vi "RTG_Host_Main.vi"() -> ()   [LabVIEW 2020]
uses:
  <vilib>/RTG/API/interface/public/State.ctl
  <vilib>/RTG/API/ip/common/host-types/Target Configuration.ctl
  <vilib>/RTG/API/ip/common/host-types/Synchronization - Host.ctl
  <vilib>/RTG/API/ip/common/host-types/Synchronization Mode - Host.ctl
  <vilib>/RTG/API/ip/common/host-types/Basic Target - Host.ctl
  <vilib>/RTG/API/ip/common/host-types/Target Motion Parameters.ctl
  <vilib>/RTG/API/ip/common/host-types/Single Target Motion Parameters.ctl
  <vilib>/RTG/API/interface/public/Coprocessor Link Status.ctl
  <vilib>/RTG/coprocessor/host/RTG Coprocessor Link Interface/Public/Coprocessor Status.ctl
  Controls/Enum/Program_Status_Enum.ctl
  Controls/Enum/RTG_Enum.ctl
  Controls/Enum/CoProcessor_Enum.ctl
  Controls/Enum/Supervisor_Enum.ctl
  Controls/Clust/RTG Clust.ctl
  <vilib>/RTG/API/interface/NI-RTG Interface.lvclass
  Controls/Clust/CoProcessor Clust.ctl
  <vilib>/RTG/coprocessor/host/RTG Coprocessor Link Interface/RTG Coprocessor Link Interface.lvclass
  Controls/Clust/RTG API Clust.ctl
  support/Options - API Mode.ctl
  support/Options - Calibration.ctl
  support/Options - Remote.ctl
  <vilib>/Utility/error.llb/Error Cluster From Error Code.vi
  <vilib>/rvi/errors/niLvFpgaAdjustHostInterfaceError.vi
  <vilib>/rvi/interface/nirviReadWriteControl/nirviReadWriteControl.xnode
  RTG Examples.lvlib
  <vilib>/RTG/API/ip/common/host-types/Host Data Types v1.lvlib
  NiFpgaLv.dll
  <vilib>/rvi/interface/Simulation/niFpgaSimulationCallBeginRW.vi
panel:
  out "CoPr":i32
  out "RTG":i32
  out "Spvsr":i32
  out "Spvsr":T1=enum."Spvsr_InitCtrls"
  out "CoPr":T2
  out "RTG":T3
  out "App Status":T4
  in  "Tab Control":T5(tab)
  in  "Instrument Names":string[](array[string])=["5831_0"]
  in  "Coprocessor Names":string[](array[string])
  in  "Center Freqeuncies (Hz)":dbl[](array[numeric])=[5500000000.0] format="%#_6p"
  in  "Reference Levels (dBm)":dbl[](array[numeric])=[0.0]
  in  "Calibrate":bool=TRUE
  in  "abort system self cal":bool
  in  "Commit HW":bool
  in  "ExtAtten":dbl[](array[numeric]) caption="External Attenuations (dB)"
  in  "OffsFreq":dbl[](array[numeric]) caption="Offset Frequencies (Hz)" format="%#_6p"
  in  "ExtDelay":dbl[](array[numeric]) caption="External Delay (s)" format="%#_6p"
  in  "mmWave Radio Heads Enable":bool[](array[boolean])
  in  "PRI (s)":dbl[](array[numeric]) format="%#_6p"
  in  "Set PRIs":bool
  out "Min Latencies (s)":dbl[](array[numeric]) format="%#_6p"
  out "Min Common Attenuations (dB)":dbl[](array[numeric])
  out "Max Common Attenuations (dB)":dbl[](array[numeric])
  out "Versions":string[](array[string])
  in  "Common Attenuation (dB)":dbl
  in  "Auto Send Software Trigger":bool
  in  "Prepend Software Trigger":bool
  in  "Device Index":i32
  in  "Target Configuration Files":path[](array[path])
  in  "Target Configuration":T6 {"rtg targets"."time offset (s)" format="%#_6p"; "rtg targets"."doppler" format="%#_6p"}
  in  "Target Motion Parameters":T10={"target motions"=[{"target enable"=FALSE, "start time offset (s)"=-1e-09, "time offset rate of change (s/s)"=0.001, "start attenuation (dB)"=0.0, "attenuation rate of change (dB/s)"=0.0, "start frequency shift (Hz)"=0.0, "frequency shift rate of change (Hz/sec)"=0.0}], "scenario duration (s)"=67.0, "configuration update rate(Hz)"=15000.0} {"configuration update rate(Hz)" format="%#_6p"; "target motions"."frequency shift rate of change (Hz/sec)" format="%#_6p"; "target motions"."start frequency shift (Hz)" format="%#_6p"; "target motions"."time offset rate of change (s/s)" format="%#_6p"; "target motions"."start time offset (s)" format="%#_6p"}
  in  "Send TrgtCfg":bool
  in  "Send Motion":bool
  in  "Send Files":bool
  in  "Start RTG":bool
  in  "Stop RTG":bool
  in  "Send SW Trigg":bool
  out "rtg link status":T12[](array[typedef])
  out "Trigger Count":i32[][](array[numeric]) caption="Device Index vs Trigger Count"
  out "RTG Status":string
  out "RTG State":T13
  out "error out":errorcluster
  out "System Time":string
  out "coproc link":T14[](array[typedef]) caption="coprocessor link status"
  in  "Exit":bool
  # "v20230901"
  # "Configuration Files and Target Motion"
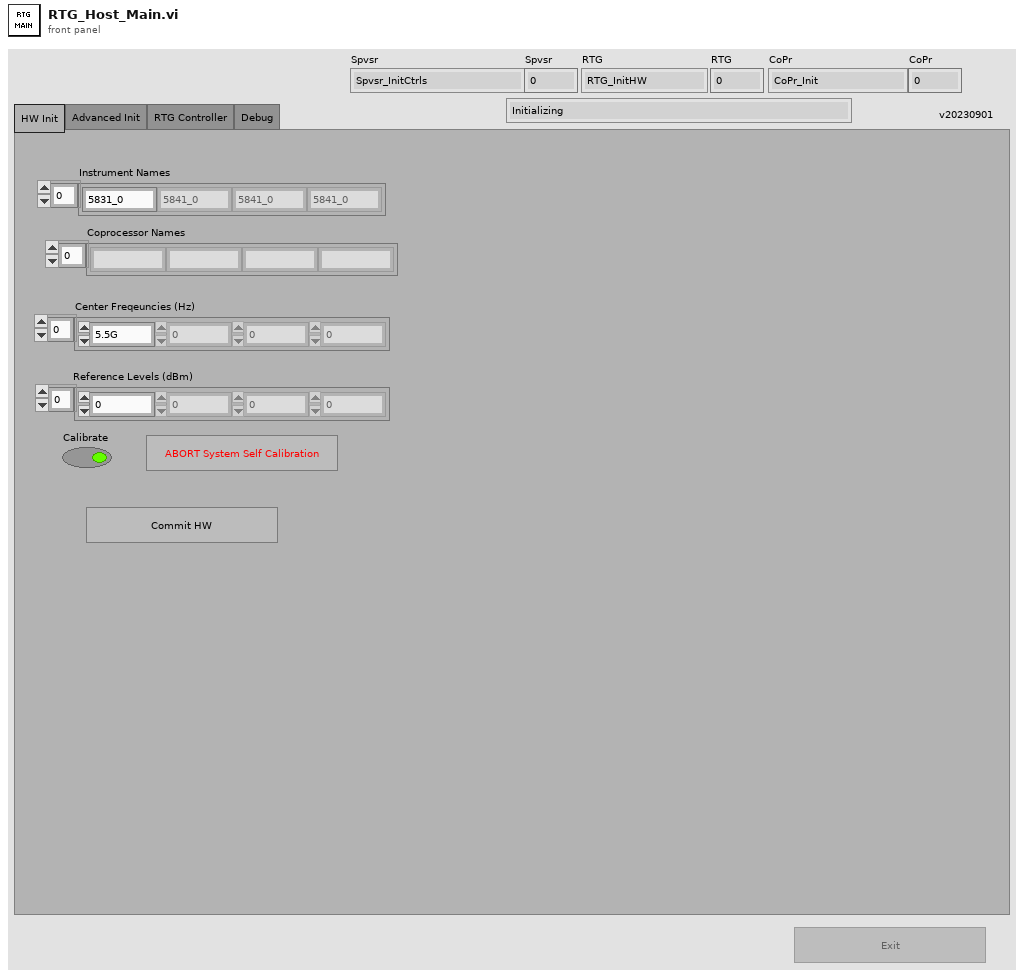
[diagram p1: front panel]
types:
  T1 = typedef "Supervisor_Enum.ctl" = enum16{"Spvsr_InitSW", "Spvsr_InitCtrls", "Spvsr_UpdtFP", "Spvsr_InitRTG", "Spvsr_StateCount", "Spvsr_Exit"}
  T2 = typedef "CoProcessor_Enum.ctl" = enum16{"CoPr_Init", "CoPr_Chk", "CoPr_Exit"}
  T3 = typedef "RTG_Enum.ctl" = enum16{"RTG_InitHW", "RTG_RefLvl", "RTG_mmWav", "RTG_Cal", "RTG_CalDone?", "RTG_ExtAtten", "RTG_GetCal", "RTG_SetPRIs", "RTG_CommAtten", "RTG_TargetSetup", "RTG_Send Files", "RTG_Send Target Cfg", "RTG_Send Motion", "RTG_Send SW Trigg", "RTG_Start", "RTG_Stop", "RTG_Chk", "RTG_Exit"}
  T4 = typedef "Program_Status_Enum.ctl" = enum16{"Initializing", "RTG Inactive", "Unconfigured", "RTG active", "Error", "Closing", "Closed"}
  T5 = enum32{"HW Init", "Advanced Init", "RTG Controller", "Debug"}
  T6 = typedef "Host Data Types v1.lvlib/Target Configuration.ctl" = cluster{"synchronization":T7, "rtg targets":T9[]}
  T7 = typedef "Host Data Types v1.lvlib/Synchronization - Host.ctl" = cluster{"synch mode":T8, "time offset (s)":dbl}
  T8 = typedef "Host Data Types v1.lvlib/Synchronization Mode - Host.ctl" = enum16{"Software Trigger", "Hardware Trigger", "Time Offset Relative to First", "Time Offset Relative to Last", "Pulse Rising Edge", "Pulse Falling Edge"}
  T9 = typedef "Host Data Types v1.lvlib/Basic Target - Host.ctl" = cluster{"time offset (s)":dbl, "attenuaton (dB)":dbl, "doppler":dbl, "target enable":bool, "relative velocity enable":bool}
  T10 = typedef "Host Data Types v1.lvlib/Target Motion Parameters.ctl" = cluster{"target motions":T11[], "scenario duration (s)":dbl, "configuration update rate(Hz)":dbl}
  T11 = typedef "Host Data Types v1.lvlib/Single Target Motion Parameters.ctl" = cluster{"target enable":bool, "start time offset (s)":dbl, "time offset rate of change (s/s)":dbl, "start attenuation (dB)":dbl, "attenuation rate of change (dB/s)":dbl, "start frequency shift (Hz)":dbl, "frequency shift rate of change (Hz/sec)":dbl}
  T12 = typedef "NI-RTG v1.lvlib/NI-RTG Interface.lvclass/Coprocessor Link Status.ctl" = cluster{"task name":string, "device name":string, "hard error":bool, "soft error":bool, "channel up":bool, "system reset":bool}
  T13 = typedef "NI-RTG v1.lvlib/NI-RTG Interface.lvclass/State.ctl" = enum16{"Idle", "Inactive", "Active", "System Self Calibration"}
  T14 = typedef "RTG Coprocessor Link Interface v1 Host.lvlib/RTG Coprocessor Link Interface.lvclass/Coprocessor Status.ctl" = cluster{"tx read count":u64, "tx read overflow":bool, "rx read count":u64, "rx read overflow":bool}
  T15 = typedef "CoProcessor Clust.ctl" = cluster{"CoPr Refs":refnum<class "RTG Coprocessor Link Interface.lvclass">[]}
  T16 = typedef "RTG Clust.ctl" = cluster{"VST_Names":string[], "OptionString":string, "RTG Ref":refnum<class "NI-RTG Interface.lvclass">, "Index":i32, "AutoSend":bool, "Prepend":bool, "state":T13}
  T17 = enum8{"Enabled", "Disabled", "Disabled and Grayed Out"}
  T18 = typedef "RTG API Clust.ctl" = cluster{"Local?":T19, "Cal":T20, "Remote":T21, "ini path":path}
  T19 = typedef "RTG Examples.lvlib/Options - API Mode.ctl" = enum16{"Local", "Remote"}
  T20 = typedef "RTG Examples.lvlib/Options - Calibration.ctl" = cluster{"enable internal loopback  ":bool, "enable overwrite cal data  ":bool, "enable save cal data           ":bool, "disable self cal range          ":bool}
  T21 = typedef "RTG Examples.lvlib/Options - Remote.ctl" = cluster{"ip address":string, "port":string, "certificate path":path, "timeout (ms)":i32}
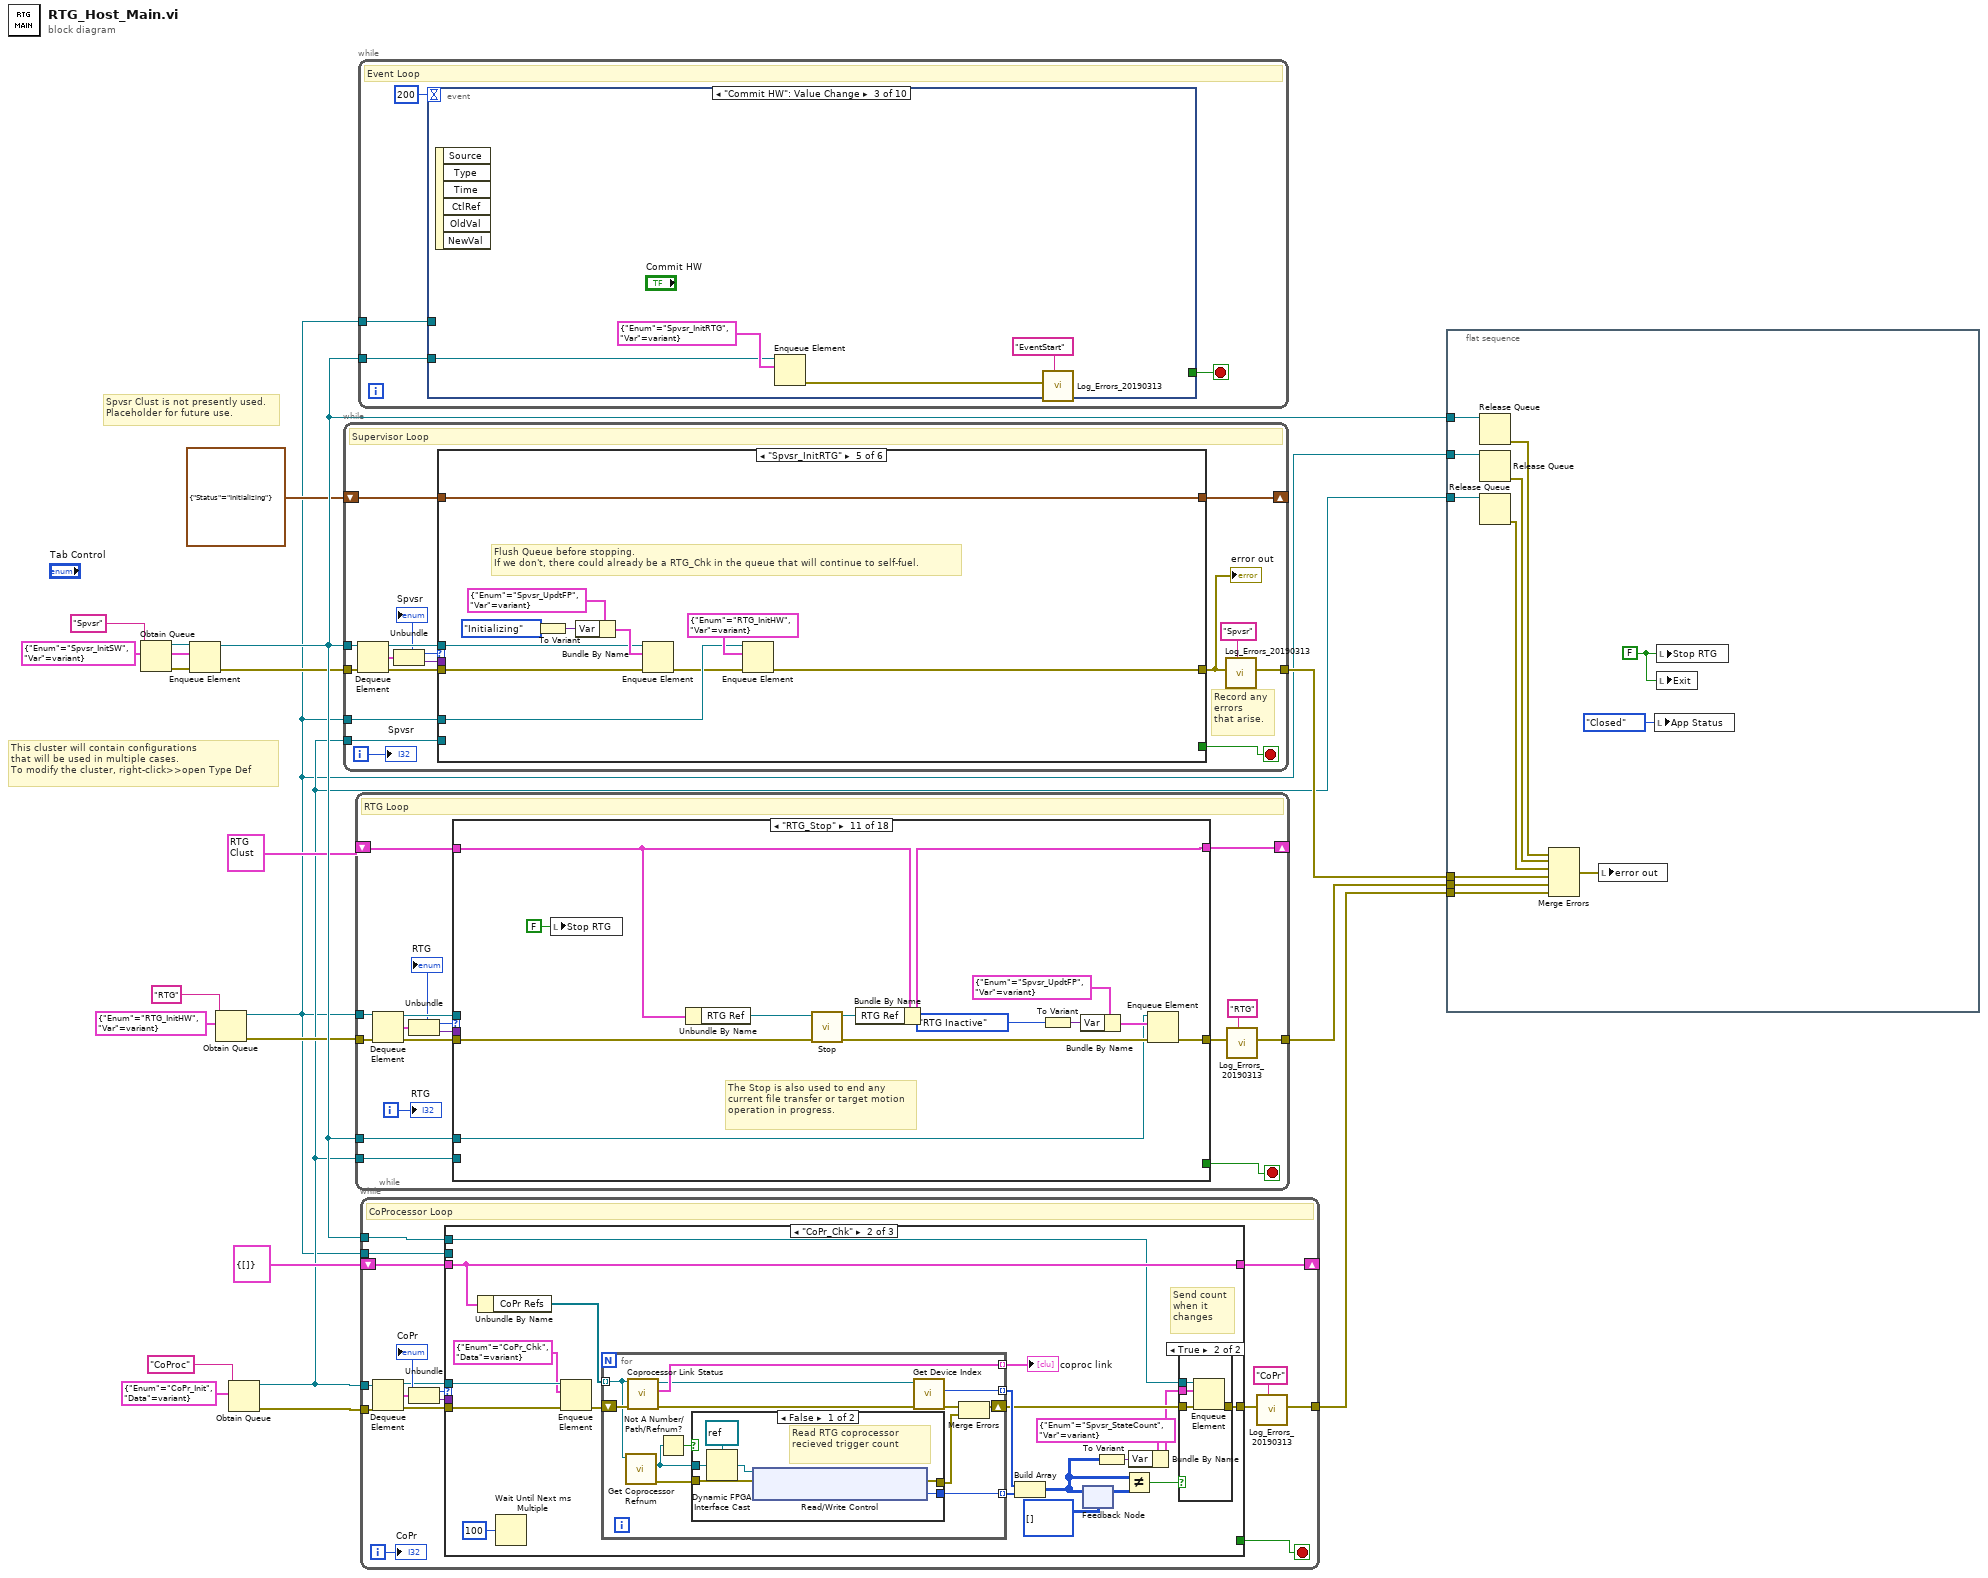
[diagram p0: block diagram]
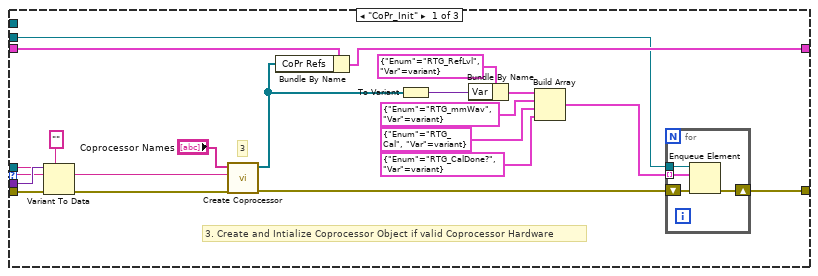
[diagram p2: hidden frame]
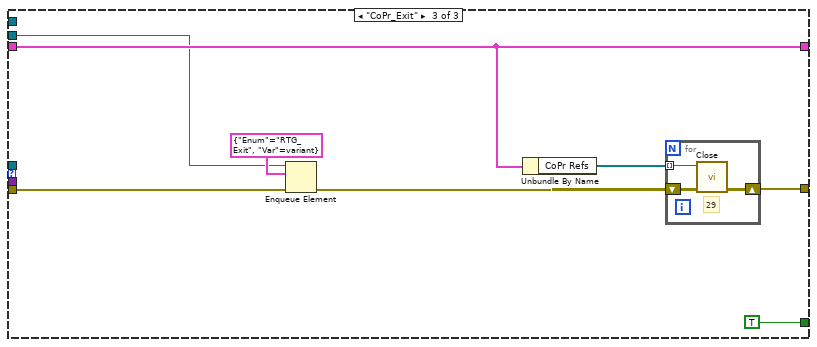
[diagram p5: hidden frame]
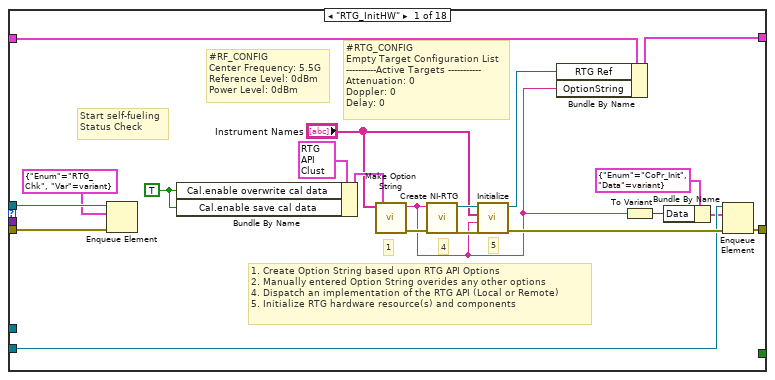
[diagram p6: hidden frame]
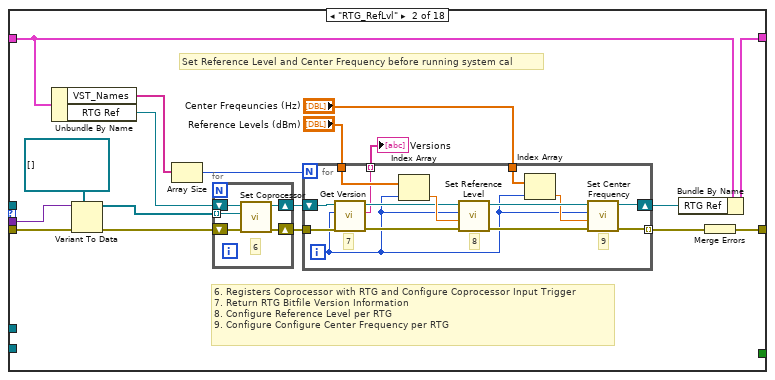
[diagram p7: hidden frame]
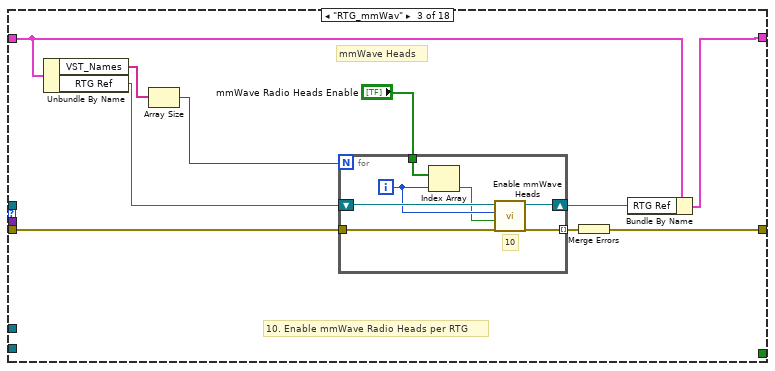
[diagram p8: hidden frame]
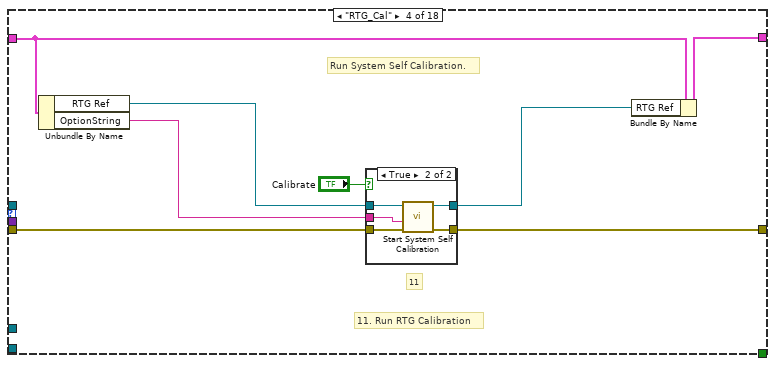
[diagram p9: hidden frame]
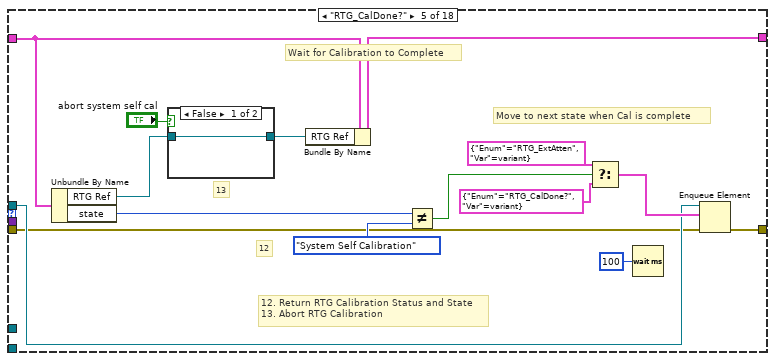
[diagram p11: hidden frame]
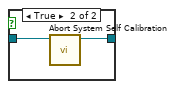
[diagram p12: hidden frame]
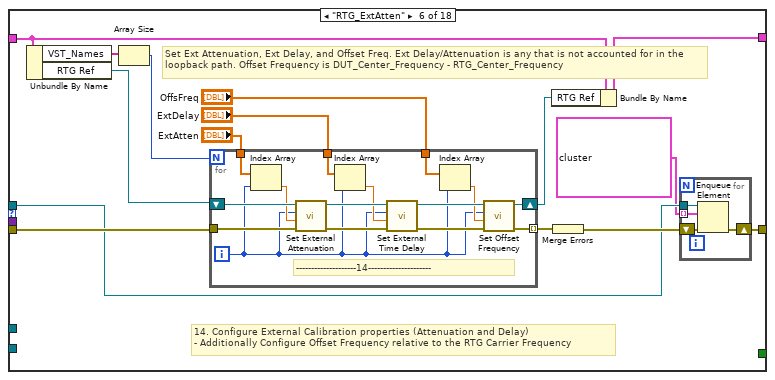
[diagram p13: hidden frame]
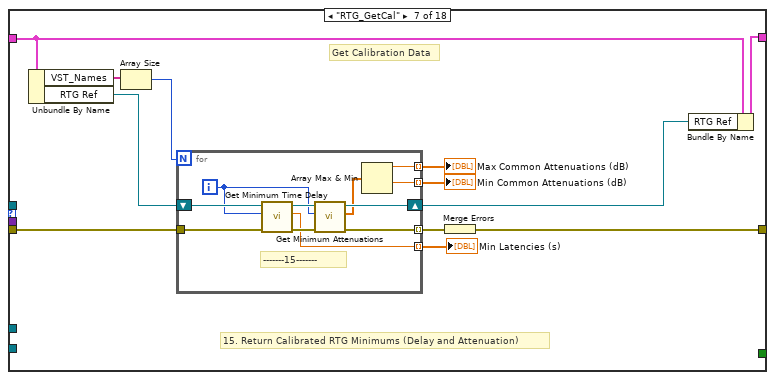
[diagram p14: hidden frame]
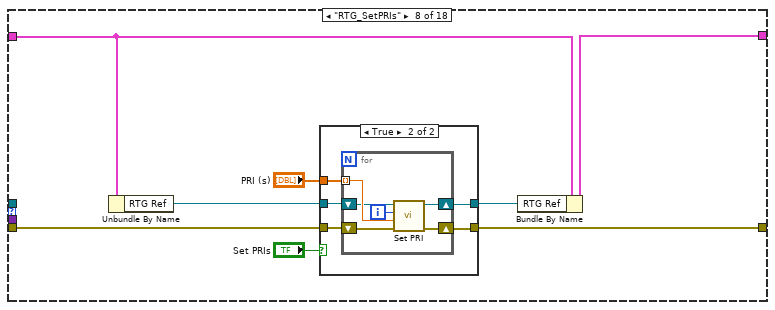
[diagram p15: hidden frame]
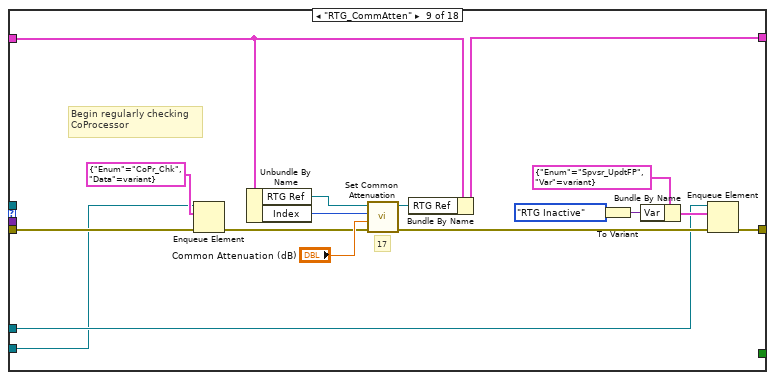
[diagram p17: hidden frame]
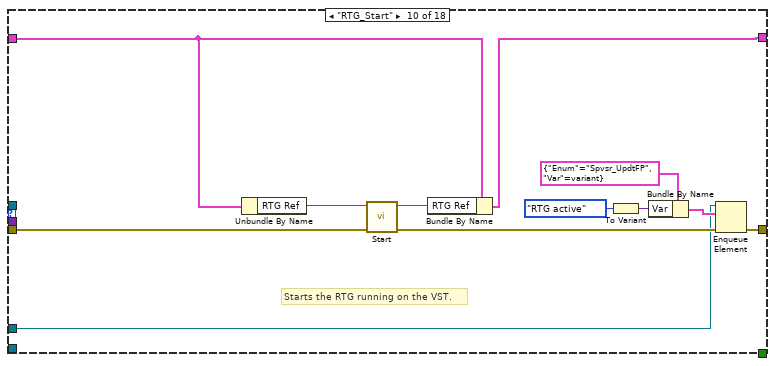
[diagram p18: hidden frame]
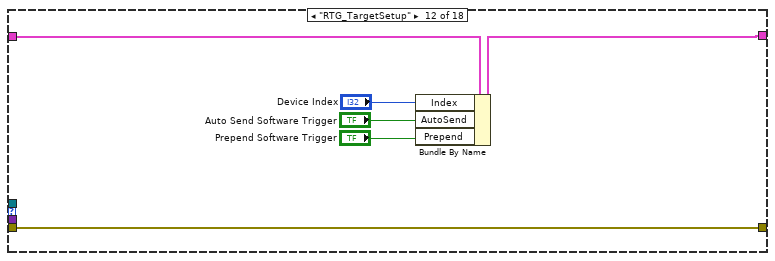
[diagram p19: hidden frame]
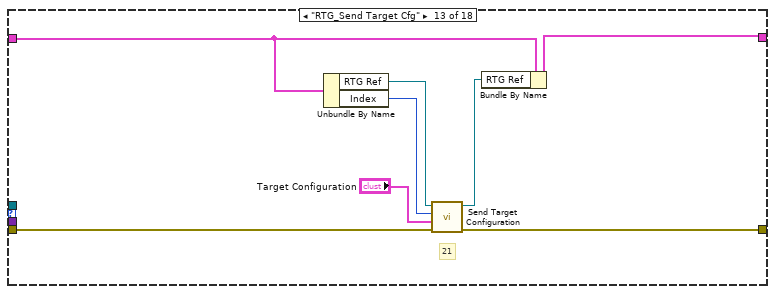
[diagram p20: hidden frame]
diagram:
  w16 = cluster{"Enum":T1, "Var":variant} {"Enum"=enum."Spvsr_InitSW", "Var"=variant}
  # "Spvsr Clust is not presently used.\nPlaceholder for future use."
  # "This cluster will contain configurations\nthat will be used in multiple cases.\nTo modify the cluster, right-click>>open Type Def"
  n1 = Obtain Queue(name (unnamed)="Spvsr", element data type=w16) -> (queue out=w17:refnum<queue>, error out=w19:errorcluster)  [unwired: 3 in, 1 out]
  n2 = Enqueue Element(queue=w17, element=w16, error in (no error)=w19) -> (queue out=w20:refnum<queue>, error out=w18:errorcluster)  [unwired: 1 in, 1 out]
  n3 = Obtain Queue(name (unnamed)="RTG", element data type=cluster{"Enum":T3, "Var":variant} {"Enum"=enum."RTG_InitHW", "Var"=variant}) -> (queue out=w1:refnum<queue>, error out=w14:errorcluster)  [unwired: 3 in, 1 out]
  n4 = Obtain Queue(name (unnamed)="CoProc", element data type=cluster{"Enum":T2, "Data":variant} {"Enum"=enum."CoPr_Init", "Data"=variant}) -> (queue out=w2:refnum<queue>, error out=w12:errorcluster)  [unwired: 3 in, 1 out]
  n5 = while {
    tunnel: w18 -> [w36]
    tunnel: w20 -> [w34]
    tunnel: w1 -> [w29]
    tunnel: [w26] -> w6
    tunnel: w2 -> [w25]
    shift-right: [w23] -> _
    shift-left: cluster{"Status":T4} {"Status"=enum."Initializing"} -> [w24]
    i -> [w21]
    stop <- w22 stop-if-true
    # "Record any\nerrors \nthat arise."
    # "Supervisor Loop"
    n6 = Dequeue Element(queue=w34, error in (no error)=w36) -> (queue out=w32:refnum<queue>, element=w33:cluster{"Enum":T1, "Var":variant}, error out=w35:errorcluster)  [unwired: 1 in, 1 out]
    n7 = Unbundle(w33) -> ("Enum"=w31:T1, "Var"=w30:variant)
    "Spvsr" <- w31
    n8 = case shown="\"Spvsr_InitRTG\"" w31 {
      tunnel: w35 -> [w47 w49 w60 w122 w128 w140]
      tunnel: w32 -> [w46 w48 _ _ w125 _]
      tunnel: w30 -> [_ _ w59 _ _ w138]
      tunnel: w29 -> [_ _ _ w120 w134 _]
      tunnel: [w44 w50 w62 w119 w126 w136] -> w27
      tunnel: w25 -> [_ _ _ w117 _ _]
      tunnel: w24 -> [w37 w55 w75 w113 w133 w141]
      tunnel: [w37 w55 w75 w113 w133 w141] -> w23
      tunnel: [_ _ _ TRUE _ _] -> w22
      frame "Spvsr_InitSW" {
        n9 = Enqueue Element(queue=w46, element=cluster{"Enum":T1, "Var":variant} {"Enum"=enum."Spvsr_InitCtrls", "Var"=variant}, error in (no error)=w47) -> (queue out=w42:refnum<queue>, error out=w43:errorcluster)  [unwired: 1 in, 1 out]
        n10 = To Variant(anything=Program_Status_Enum."Initializing" ("Status")) -> (Variant=w39:variant)
        n11 = Bundle By Name(cluster=cluster{"Enum":T1, "Var":variant} {"Enum"=enum."Spvsr_UpdtFP", "Var"=variant}, "Var"=w39) -> (w38:cluster{"Enum":T1, "Var":variant})
        n12 = Enqueue Element(queue=w42, element=w38, error in (no error)=w43) -> (error out=w44:errorcluster)  [unwired: 1 in, 2 out]
      }
      frame "Spvsr_InitCtrls" {
        w56 = FALSE ("Exit")
        n13 = To Variant(anything=Program_Status_Enum."Unconfigured" ("Status")) -> (Variant=w54:variant)
        n14 = Bundle By Name(cluster=cluster{"Enum":T1, "Var":variant} {"Enum"=enum."Spvsr_UpdtFP", "Var"=variant}, "Var"=w54) -> (w52:cluster{"Enum":T1, "Var":variant})
        n15 = Enqueue Element(queue=w48, element=w52, error in (no error)=w49) -> (error out=w50:errorcluster)  [unwired: 1 in, 2 out]
        n16 = local write "Exit"(w56) -> ()
        n17 = local write "Stop RTG"(w56) -> ()
      }
      frame "Spvsr_UpdtFP" {
        n18 = Variant To Data(error in=w60, type=Program_Status_Enum."Closed" ("App Status"), Variant=w59) -> (data=w57:T4, error out=w61:errorcluster)
        "App Status" <- w57
        n19 = case shown="\"Unconfigured\"" w57 {
          tunnel: [T17."Disabled and Grayed Out" ("Disabled") T17."Enabled" ("Disabled") T17."Disabled and Grayed Out" ("Disabled") T17."Disabled and Grayed Out" ("Disabled") T17."Enabled" ("Disabled") T17."Disabled and Grayed Out" ("Disabled")] -> w68
          tunnel: [T17."Disabled and Grayed Out" ("Disabled") T17."Enabled" ("Disabled") T17."Disabled and Grayed Out" ("Disabled") T17."Disabled and Grayed Out" ("Disabled") T17."Disabled and Grayed Out" ("Disabled") T17."Enabled" ("Disabled")] -> w67
          tunnel: [T17."Enabled" ("Disabled") T17."Enabled" ("Disabled") T17."Disabled and Grayed Out" ("Disabled") T17."Enabled" ("Disabled") T17."Enabled" ("Disabled") T17."Enabled" ("Disabled")] -> w66
          tunnel: [T17."Disabled and Grayed Out" ("Disabled") T17."Disabled and Grayed Out" ("Disabled") T17."Disabled and Grayed Out" ("Disabled") T17."Disabled and Grayed Out" ("Disabled") T17."Disabled and Grayed Out" ("Disabled") T17."Enabled" ("Disabled")] -> w65
          tunnel: [T17."Disabled and Grayed Out" ("Disabled") T17."Disabled and Grayed Out" ("Disabled") T17."Disabled and Grayed Out" ("Disabled") T17."Disabled and Grayed Out" ("Disabled") T17."Disabled and Grayed Out" ("Disabled") T17."Enabled" ("Disabled")] -> w64
          tunnel: [T17."Disabled and Grayed Out" ("Disabled") T17."Disabled and Grayed Out" ("Disabled") T17."Disabled and Grayed Out" ("Disabled") T17."Disabled and Grayed Out" ("Disabled") T17."Disabled and Grayed Out" ("Disabled") T17."Enabled" ("Disabled")] -> w63
          frame "Unconfigured" {
          }
          frame "Error" {
          }
          frame "Closing", "Closed" {
          }
          frame "Initializing" {
          }
          frame "RTG Inactive" {
          }
          frame "RTG active" {
          }
        }
        n20 = property on="Start RTG" class="Bool"(error in=w61, "DisabledEnum"=w68) -> (error out=w69:errorcluster)  [unwired: 1 in, 1 out]
        n21 = property on="Stop RTG" class="Bool (strict)"("DisabledEnum"=w67) -> (error out=w70:errorcluster)  [unwired: 2 in, 1 out]
        n22 = property on="Exit" class="Bool (strict)"("DisabledEnum"=w66) -> (error out=w71:errorcluster)  [unwired: 2 in, 1 out]
        n23 = property on="Send TrgtCfg" class="Bool"("DisabledEnum"=w65) -> (error out=w72:errorcluster)  [unwired: 2 in, 1 out]
        n24 = property on="Send Motion" class="Bool"("DisabledEnum"=w64) -> (error out=w73:errorcluster)  [unwired: 2 in, 1 out]
        n25 = property on="Send Files" class="Bool"("DisabledEnum"=w63) -> (error out=w74:errorcluster)  [unwired: 2 in, 1 out]
        n26 = Merge Errors(w69, w70, w71, w72, w73, w74) -> (w62:errorcluster)
      }
      frame "Spvsr_Exit" {
        # "RTG Exit is called from Coprocesor Exit\nto prevent a race condition"
        # "Flush Queue before stopping.\nIf we don't, there could already be a RTG_Chk in the queue that will continue to self-fuel."
        n27 = Flush Queue(queue=w120, error in (no error)=w122) -> (queue out=w121:refnum<queue>, error out=w123:errorcluster)  [unwired: 1 out]
        n28 = Enqueue Element(queue=w121, element=cluster{"Enum":T3, "Var":variant} {"Enum"=enum."RTG_Stop", "Var"=variant}, error in (no error)=w123) -> (error out=w115:errorcluster)  [unwired: 1 in, 2 out]
        n29 = Flush Queue(queue=w117, error in (no error)=w115) -> (queue out=w116:refnum<queue>, error out=w114:errorcluster)  [unwired: 1 out]
        n30 = Enqueue Element(queue=w116, element=cluster{"Enum":T2, "Data":variant} {"Enum"=enum."CoPr_Exit", "Data"=variant}, error in (no error)=w114) -> (error out=w119:errorcluster)  [unwired: 1 in, 2 out]
      }
      frame "Spvsr_InitRTG" {
        # "Flush Queue before stopping.\nIf we don't, there could already be a RTG_Chk in the queue that will continue to self-fuel."
        n31 = To Variant(anything=Program_Status_Enum."Initializing" ("Status")) -> (Variant=w132:variant)
        n32 = Bundle By Name(cluster=cluster{"Enum":T1, "Var":variant} {"Enum"=enum."Spvsr_UpdtFP", "Var"=variant}, "Var"=w132) -> (w130:cluster{"Enum":T1, "Var":variant})
        n33 = Enqueue Element(queue=w125, element=w130, error in (no error)=w128) -> (error out=w127:errorcluster)  [unwired: 1 in, 2 out]
        n34 = Enqueue Element(queue=w134, element=cluster{"Enum":T3, "Var":variant} {"Enum"=enum."RTG_InitHW", "Var"=variant}, error in (no error)=w127) -> (error out=w126:errorcluster)  [unwired: 1 in, 2 out]
      }
      frame "Spvsr_StateCount" {
        # "Making this value available to the rest of the program."
        n35 = Variant To Data(error in=w140, type=i32[][] [] ("appended array"), Variant=w138) -> (data=→"Trigger Count":i32[][], error out=w136:errorcluster)
      }
    }
    "error out" <- w27
    n36 = call "Log_Errors_20190313.vi"("LoopName"="Spvsr", "error in"=w27) -> ("error out"=w26:errorcluster)  [unwired: 9 in]
    "Spvsr" <- w21
  }
  n37 = while {
    tunnel: w14 -> [w157]
    shift-right: [w149] -> _
    shift-left: T16 {"VST_Names"=["5841_0"], "OptionString"="", "RTG Ref"=refnum, "Index"=0, "AutoSend"=FALSE, "Prepend"=FALSE, "state"=enum."Idle"} ("DAQ Clust") -> [w150]
    tunnel: [w147] -> w5
    tunnel: w2 -> [w146]
    tunnel: w1 -> [w143]
    tunnel: w20 -> [w142]
    i -> [w144]
    stop <- w145 stop-if-true
    # "RTG Loop"
    n38 = Dequeue Element(queue=w143, error in (no error)=w157) -> (queue out=w154:refnum<queue>, element=w155:cluster{"Enum":T3, "Var":variant}, error out=w156:errorcluster)  [unwired: 1 in, 1 out]
    n39 = Unbundle(w155) -> ("Enum"=w153:T3, "Var"=w152:variant)
    "RTG" <- w153
    n40 = case shown="\"RTG_Stop\"" w153 {
      tunnel: w156 -> [w160 w186 w219 w236 w248 w274 w303 w325 w344 w371 w380 w390 w397 w405 w434 w461 w473 w483]
      tunnel: w154 -> [w159 _ _ _ w251 w266 _ _ _ _ _ _ _ _ _ _ w472 _]
      tunnel: w152 -> [_ w183 _ _ _ _ _ _ _ _ _ _ _ _ _ _ _ _]
      tunnel: w150 -> [w177 w180 w215 w239 w261 w279 w309 w329 w359 w367 w383 w388 w394 w412 w441 w463 w478 w480]
      tunnel: [w176 w179 w216 w238 w260 w278 w310 w328 w358 w368 w384 w389 w393 w411 w440 w462 w477 w480] -> w149
      tunnel: [w166 w181 w218 w235 w250 w267 w302 w324 w350 w361 w373 w390 w396 w404 w433 w460 w467 w482] -> w148
      tunnel: w146 -> [w165 _ _ _ _ _ _ _ w343 _ _ _ _ _ _ _ _ _]
      tunnel: [_ _ _ _ _ _ _ _ _ _ _ _ _ _ _ _ _ TRUE] -> w145
      tunnel: w142 -> [_ _ _ _ _ _ _ _ w347 w360 w372 _ _ _ _ _ _ _]
      frame "RTG_InitHW" {
        w175 = TRUE ("Calibration Options.enable overwrite cal data")
        # "Start self-fueling\nStatus Check"
        # "1. Create Option String based upon RTG API Options\n2. Manually entered Option String overides any other options\n4. Dispatch an implementation of the RTG API (Local or Remote)\n5. Initialize RTG hardware resource(s) and components"
        # "#RTG_CONFIG\nEmpty Target Configuration List\n----------Active Targets -----------\nAttenuation: 0\nDoppler: 0\nDelay: 0"
        # "#RF_CONFIG\nCenter Frequency: 5.5G\nReference Level: 0dBm\nPower Level: 0dBm"
        # "4"
        # "1"
        # "5"
        n41 = Enqueue Element(queue=w159, element=cluster{"Enum":T3, "Var":variant} {"Enum"=enum."RTG_Chk", "Var"=variant}, error in (no error)=w160) -> ()  [unwired: 1 in, 3 out]
        n42 = Bundle By Name(cluster=T18 {"Local?"=enum."Local", "Cal"={"enable internal loopback  "=FALSE, "enable overwrite cal data  "=FALSE, "enable save cal data           "=FALSE, "disable self cal range          "=FALSE}, "Remote"={"ip address"="", "port"="50052", "certificate path"=path "", "timeout (ms)"=15000}, "ini path"=path ""} ("RTG API Options"), "Cal.enable overwrite cal data"=w175, "Cal.enable save cal data"=w175) -> (w174:T18)
        n43 = call "Make Option String.vi"("RTG API Options"=w174, "instrument names"="Instrument Names") -> ("error out"=w173:errorcluster, "option string"=w163:string)  [unwired: 8 in]
        n44 = call <vilib>:"Create NI-RTG.vi"("error in"=w173, "option string"=w163) -> ("error out"=w171:errorcluster, "NI-RTG Interface out"=w170:refnum<class "NI-RTG Interface.lvclass">)  [unwired: 8 in]
        n45 = call-dynamic "Initialize.vi"("error in"=w171, "option string"=w163, "instrument names"="Instrument Names", "ni-rtg interface"=w170) -> ("error out"=w167:errorcluster, "ni-rtg interface out"=w168:refnum<class "NI-RTG Interface.lvclass">)  [unwired: 6 in]
        n46 = Bundle By Name(cluster=w177, "RTG Ref"=w168, "OptionString"=w163) -> (w176:T16)
        n47 = To Variant(anything=w163) -> (Variant=w162:variant)
        n48 = Bundle By Name(cluster=cluster{"Enum":T2, "Data":variant} {"Enum"=enum."CoPr_Init", "Data"=variant}, "Data"=w162) -> (w161:cluster{"Enum":T2, "Data":variant})
        n49 = Enqueue Element(queue=w165, element=w161, error in (no error)=w167) -> (error out=w166:errorcluster)  [unwired: 1 in, 2 out]
      }
      frame "RTG_RefLvl" {
        # "6. Registers Coprocessor with RTG and Configure Coprocessor Input Trigger\n7. Return RTG Bitfile Version Information\n8. Configure Reference Level per RTG\n9. Configure Configure Center Frequency per RTG"
        # "Set Reference Level and Center Frequency before running system cal"
        n50 = Unbundle By Name(w180) -> ("VST_Names"=w188:string[], "RTG Ref"=w189:refnum<class "NI-RTG Interface.lvclass">)
        n51 = Variant To Data(error in=w186, type=refnum<class "RTG Coprocessor Link Interface.lvclass">[] [] ("rtg coprocessor links"), Variant=w183) -> (data=w182:refnum<class "RTG Coprocessor Link Interface.lvclass">[], error out=w185:errorcluster)
        n52 = Array Size(array=w188) -> (size(s)=w187:i32)
        n53 = for {
          shift-right: [w214] -> w193
          shift-left: w185 -> [w212]
          shift-right: [w213] -> w194
          shift-left: w189 -> [w211]
          tunnel: w182 -> [w210] mode=indexing
          # "6"
          n54 = call-dynamic "Set Coprocessor.vi"("error in"=w212, "rtg coprocessor link interface"=w210, "rtg api interface"=w211) -> ("error out"=w214:errorcluster, "rtg api interface out"=w213:refnum<class "NI-RTG Interface.lvclass">)  [unwired: 7 in]
        }
        n55 = for {
          N: w187 -> [_]
          tunnel: w193 -> [w199]
          tunnel: "Reference Levels (dBm)" -> [w207]
          tunnel: "Center Freqeuncies (Hz)" -> [w205]
          shift-right: [w203] -> w178
          shift-left: w194 -> [w201]
          tunnel: [w202] -> w192 mode=indexing
          tunnel: [w196] -> w195 mode=indexing
          i -> [w197]
          # "9"
          # "8"
          # "7"
          n56 = call-dynamic "Get Version.vi"("error in"=w199, "device index (0)"=w197, "NI-RTG Interface in"=w201) -> ("error out"=w198:errorcluster, "version"=w196:string, "NI-RTG Interface out"=w200:refnum<class "NI-RTG Interface.lvclass">)  [unwired: 6 in]
          n57 = Index Array(array=w207, index=w197) -> (element=w206:dbl)
          n58 = call-dynamic "Set Reference Level.vi"("error in"=w198, "reference level (dBm)"=w206, "device index (0)"=w197, "rtg api interface"=w200) -> ("error out"=w208:errorcluster, "rtg api interface out"=w209:refnum<class "NI-RTG Interface.lvclass">)  [unwired: 6 in]
          n59 = Index Array(array=w205, index=w197) -> (element=w204:dbl)
          n60 = call-dynamic "Set Center Frequency.vi"("error in"=w208, "center frequency (Hz)"=w204, "device index (0)"=w197, "rtg api interface"=w209) -> ("error out"=w202:errorcluster, "rtg api interface out"=w203:refnum<class "NI-RTG Interface.lvclass">)  [unwired: 6 in]
        }
        "Versions" <- w195
        n61 = Bundle By Name(cluster=w180, "RTG Ref"=w178) -> (w179:T16)
        n62 = Merge Errors(w192) -> (w181:errorcluster)
      }
      frame "RTG_mmWav" {
        # "10. Enable mmWave Radio Heads per RTG"
        # "mmWave Heads"
        n63 = Unbundle By Name(w215) -> ("VST_Names"=w224:string[], "RTG Ref"=w221:refnum<class "NI-RTG Interface.lvclass">)
        n64 = Array Size(array=w224) -> (size(s)=w220:i32)
        n65 = for {
          N: w220 -> [_]
          shift-right: [w228] -> w217
          shift-left: w221 -> [w229]
          tunnel: w219 -> [w231]
          tunnel: [w230] -> w222 mode=indexing
          tunnel: "mmWave Radio Heads Enable" -> [w227]
          i -> [w226]
          # "10"
          n66 = Index Array(array=w227, index=w226) -> (element=w225:bool)
          n67 = call-dynamic "Enable mmWave Heads.vi"("error in"=w231, "enable mmWave"=w225, "device index (0)"=w226, "ni-rtg interface"=w229) -> ("error out"=w230:errorcluster, "ni-rtg interface out"=w228:refnum<class "NI-RTG Interface.lvclass">)  [unwired: 6 in]
        }
        n68 = Merge Errors(w222) -> (w218:errorcluster)
        n69 = Bundle By Name(cluster=w215, "RTG Ref"=w217) -> (w216:T16)
      }
      frame "RTG_Cal" {
        # "11"
        # "11. Run RTG Calibration"
        # "Run System Self Calibration."
        n70 = Unbundle By Name(w239) -> ("RTG Ref"=w234:refnum<class "NI-RTG Interface.lvclass">, "OptionString"=w232:string)
        n71 = case shown="True" "Calibrate" {
          tunnel: w234 -> [w241 w246]
          tunnel: w236 -> [w240 w245]
          tunnel: [w241 w244] -> w233
          tunnel: [w240 w243] -> w235
          tunnel: w232 -> [_ w242]
          frame False {
          }
          frame True {
            n72 = call-dynamic "Start System Self Calibration.vi"("error in"=w245, "option string"=w242, "rtg api interface"=w246) -> ("error out"=w243:errorcluster, "rtg api interface out"=w244:refnum<class "NI-RTG Interface.lvclass">)  [unwired: 7 in]
          }
        }
        n73 = Bundle By Name(cluster=w239, "RTG Ref"=w233) -> (w238:T16)
      }
      frame "RTG_CalDone?" {
        # "Move to next state when Cal is complete"
        # "13"
        # "12"
        # "12. Return RTG Calibration Status and State\n13. Abort RTG Calibration"
        # "Wait for Calibration to Complete"
        n74 = Unbundle By Name(w261) -> ("RTG Ref"=w259:refnum<class "NI-RTG Interface.lvclass">, "state"=w247:T13)
        n75 = case shown="False" "abort system self cal" {
          tunnel: w259 -> [w262 w264]
          tunnel: [w262 w263] -> w249
          frame False {
          }
          frame True {
            n76 = call-dynamic "Abort System Self Calibration.vi"("rtg-api interface"=w264) -> ("rtg-api interface out"=w263:refnum<class "NI-RTG Interface.lvclass">)  [unwired: 9 in, 1 out]
          }
        }
        n77 = Bundle By Name(cluster=w261, "RTG Ref"=w249) -> (w260:T16)
        n78 = Not Equal?(x=w247, y=State."System Self Calibration") -> (x != y?=w252:bool)
        n79 = Select(t=cluster{"Enum":T3, "Var":variant} {"Enum"=enum."RTG_ExtAtten", "Var"=variant} ("element"), s=w252, f=cluster{"Enum":T3, "Var":variant} {"Enum"=enum."RTG_CalDone?", "Var"=variant} ("element")) -> (s? t:f=w255:cluster{"Enum":T3, "Var":variant})
        n80 = Wait (ms)(milliseconds to wait=u32 100) -> ()  [unwired: 1 out]
        n81 = Enqueue Element(queue=w251, element=w255, error in (no error)=w248) -> (error out=w250:errorcluster)  [unwired: 1 in, 2 out]
      }
      frame "RTG_ExtAtten" {
        # "Set Ext Attenuation, Ext Delay, and Offset Freq. Ext Delay/Attenuation is any that is not accounted for in the loopback path. Offset Frequency is DUT_Center_Frequency - RTG_Center_Frequency"
        # "14. Configure External Calibration properties (Attenuation and Delay)\n- Additionally Configure Offset Frequency relative to the RTG Carrier Frequency"
        n82 = Unbundle By Name(w279) -> ("VST_Names"=w277:string[], "RTG Ref"=w270:refnum<class "NI-RTG Interface.lvclass">)
        n83 = Array Size(array=w277) -> (size(s)=w271:i32)
        n84 = for {
          N: w271 -> [_]
          shift-right: [w288] -> w269
          shift-left: w270 -> [w298]
          tunnel: "ExtAtten" -> [w296]
          tunnel: "ExtDelay" -> [w294]
          tunnel: [w290] -> w273 mode=indexing
          tunnel: w274 -> [w287]
          tunnel: "OffsFreq" -> [w286]
          i -> [w284]
          # "--------------------14---------------------"
          n85 = Index Array(array=w296, index=w284) -> (element=w295:dbl)
          n86 = call-dynamic "Set External Attenuation.vi"("error in"=w287, "external attenuation (dB)"=w295, "device index (0)"=w284, "rtg api interface"=w298) -> ("error out"=w292:errorcluster, "rtg api interface out"=w297:refnum<class "NI-RTG Interface.lvclass">)  [unwired: 6 in]
          n87 = Index Array(array=w294, index=w284) -> (element=w293:dbl)
          n88 = call-dynamic "Set External Time Delay.vi"("error in"=w292, "delay (s)"=w293, "device index (0)"=w284, "rtg api interface"=w297) -> ("error out"=w291:errorcluster, "rtg api interface out"=w289:refnum<class "NI-RTG Interface.lvclass">)  [unwired: 6 in]
          n89 = Index Array(array=w286, index=w284) -> (element=w285:dbl)
          n90 = call-dynamic "Set Offset Frequency.vi"("error in"=w291, "offset frequency (Hz)"=w285, "device index (0)"=w284, "NI-RTG Interface in"=w289) -> ("error out"=w290:errorcluster, "NI-RTG Interface out"=w288:refnum<class "NI-RTG Interface.lvclass">)  [unwired: 6 in]
        }
        n91 = Bundle By Name(cluster=w279, "RTG Ref"=w269) -> (w278:T16)
        n92 = Merge Errors(w273) -> (w268:errorcluster)
        n93 = for {
          tunnel: w266 -> [w281]
          tunnel: cluster{"Enum":T3, "Var":variant}[] [{"Enum"=enum."RTG_GetCal", "Var"=variant}, {"Enum"=enum."RTG_SetPRIs", "Var"=variant}, {"Enum"=enum."RTG_CommAtten", "Var"=variant}] -> [w280] mode=indexing
          shift-right: [w282] -> w267
          shift-left: w268 -> [w283]
          n94 = Enqueue Element(queue=w281, element=w280, error in (no error)=w283) -> (error out=w282:errorcluster)  [unwired: 1 in, 2 out]
        }
      }
      frame "RTG_GetCal" {
        # "15. Return Calibrated RTG Minimums (Delay and Attenuation)"
        # "Get Calibration Data"
        n95 = Unbundle By Name(w309) -> ("VST_Names"=w308:string[], "RTG Ref"=w300:refnum<class "NI-RTG Interface.lvclass">)
        n96 = Array Size(array=w308) -> (size(s)=w301:i32)
        n97 = for {
          N: w301 -> [_]
          tunnel: w303 -> [w321]
          tunnel: [w318] -> w304 mode=indexing
          shift-right: [w316] -> w299
          shift-left: w300 -> [w319]
          tunnel: [w315] -> w307 mode=indexing
          tunnel: [w313] -> w305 mode=indexing
          tunnel: [w312] -> w306 mode=indexing
          i -> [w311]
          # "-------15-------"
          n98 = call-dynamic "Get Minimum Time Delay.vi"("error in"=w321, "device index (0)"=w311, "rtg api interface"=w319) -> ("error out"=w320:errorcluster, "delay (s)"=w315:dbl, "rtg api interface out"=w317:refnum<class "NI-RTG Interface.lvclass">)  [unwired: 5 in, 1 out]
          n99 = call-dynamic "Get Minimum Attenuations.vi"("error in"=w320, "device index (0)"=w311, "rtg api interface"=w317) -> ("error out"=w318:errorcluster, "attenuations (dB)"=w314:dbl[], "rtg api interface out"=w316:refnum<class "NI-RTG Interface.lvclass">)  [unwired: 5 in, 1 out]
          n100 = Array Max & Min(array=w314) -> (max value=w313:dbl, min value=w312:dbl)  [unwired: 2 out]
        }
        "Max Common Attenuations (dB)" <- w305
        "Min Common Attenuations (dB)" <- w306
        "Min Latencies (s)" <- w307
        n101 = Merge Errors(w304) -> (w302:errorcluster)
        n102 = Bundle By Name(cluster=w309, "RTG Ref"=w299) -> (w310:T16)
      }
      frame "RTG_SetPRIs" {
        n103 = Unbundle By Name(w329) -> ("RTG Ref"=w323:refnum<class "NI-RTG Interface.lvclass">)
        n104 = case shown="True" "Set PRIs" {
          tunnel: w323 -> [w331 w333]
          tunnel: [w331 w335] -> w322
          tunnel: w325 -> [w330 w332]
          tunnel: [w330 w334] -> w324
          tunnel: "PRI (s)" -> [_ w336]
          frame False {
          }
          frame True {
            n105 = for {
              tunnel: w336 -> [w342] mode=indexing
              shift-right: [w340] -> w335
              shift-left: w333 -> [w338]
              shift-right: [w339] -> w334
              shift-left: w332 -> [w337]
              i -> [w341]
              n106 = call-dynamic "Set PRI.vi"("error in"=w337, "pri (s)"=w342, "device index (0)"=w341, "NI-RTG Interface in"=w338) -> ("error out"=w339:errorcluster, "NI-RTG Interface out"=w340:refnum<class "NI-RTG Interface.lvclass">)  [unwired: 6 in]
            }
          }
        }
        n107 = Bundle By Name(cluster=w329, "RTG Ref"=w322) -> (w328:T16)
      }
      frame "RTG_CommAtten" {
        # "Begin regularly checking\nCoProcessor"
        # "17"
        n108 = Enqueue Element(queue=w343, element=cluster{"Enum":T2, "Data":variant} {"Enum"=enum."CoPr_Chk", "Data"=variant}, error in (no error)=w344) -> (error out=w345:errorcluster)  [unwired: 1 in, 2 out]
        n109 = Unbundle By Name(w359) -> ("RTG Ref"=w356:refnum<class "NI-RTG Interface.lvclass">, "Index"=w355:i32)
        n110 = call-dynamic "Set Common Attenuation.vi"("error in"=w345, "attenuation (dB)"="Common Attenuation (dB)", "device index (0)"=w355, "rtg api interface"=w356) -> ("error out"=w351:errorcluster, "rtg api interface out"=w354:refnum<class "NI-RTG Interface.lvclass">)  [unwired: 5 in, 1 out]
        n111 = Bundle By Name(cluster=w359, "RTG Ref"=w354) -> (w358:T16)
        n112 = To Variant(anything=Program_Status_Enum."RTG Inactive" ("Status")) -> (Variant=w348:variant)
        n113 = Bundle By Name(cluster=cluster{"Enum":T1, "Var":variant} {"Enum"=enum."Spvsr_UpdtFP", "Var"=variant}, "Var"=w348) -> (w352:cluster{"Enum":T1, "Var":variant})
        n114 = Enqueue Element(queue=w347, element=w352, error in (no error)=w351) -> (error out=w350:errorcluster)  [unwired: 1 in, 2 out]
      }
      frame "RTG_Start" {
        # "Starts the RTG running on the VST."
        n115 = Unbundle By Name(w367) -> ("RTG Ref"=w370:refnum<class "NI-RTG Interface.lvclass">)
        n116 = call-dynamic "Start.vi"("error in"=w371, "rtg api interface"=w370) -> ("error out"=w362:errorcluster, "rtg api interface out"=w369:refnum<class "NI-RTG Interface.lvclass">)  [unwired: 8 in]
        n117 = Bundle By Name(cluster=w367, "RTG Ref"=w369) -> (w368:T16)
        n118 = To Variant(anything=Program_Status_Enum."RTG active" ("Status")) -> (Variant=w363:variant)
        n119 = Bundle By Name(cluster=cluster{"Enum":T1, "Var":variant} {"Enum"=enum."Spvsr_UpdtFP", "Var"=variant}, "Var"=w363) -> (w365:cluster{"Enum":T1, "Var":variant})
        n120 = Enqueue Element(queue=w360, element=w365, error in (no error)=w362) -> (error out=w361:errorcluster)  [unwired: 1 in, 2 out]
      }
      frame "RTG_Stop" {
        # "The Stop is also used to end any current file transfer or target motion operation in progress."
        n121 = local write "Stop RTG"(FALSE ("Stop RTG")) -> ()
        n122 = Unbundle By Name(w383) -> ("RTG Ref"=w382:refnum<class "NI-RTG Interface.lvclass">)
        n123 = call-dynamic "Stop.vi"("error in"=w380, "rtg api interface"=w382) -> ("error out"=w374:errorcluster, "rtg api interface out"=w381:refnum<class "NI-RTG Interface.lvclass">)  [unwired: 8 in]
        n124 = Bundle By Name(cluster=w383, "RTG Ref"=w381) -> (w384:T16)
        n125 = To Variant(anything=Program_Status_Enum."RTG Inactive" ("Status")) -> (Variant=w375:variant)
        n126 = Bundle By Name(cluster=cluster{"Enum":T1, "Var":variant} {"Enum"=enum."Spvsr_UpdtFP", "Var"=variant}, "Var"=w375) -> (w377:cluster{"Enum":T1, "Var":variant})
        n127 = Enqueue Element(queue=w372, element=w377, error in (no error)=w374) -> (error out=w373:errorcluster)  [unwired: 1 in, 2 out]
      }
      frame "RTG_TargetSetup" {
        n128 = Bundle By Name(cluster=w388, "Index"="Device Index", "AutoSend"="Auto Send Software Trigger", "Prepend"="Prepend Software Trigger") -> (w389:T16)
      }
      frame "RTG_Send Target Cfg" {
        # "21"
        n129 = Unbundle By Name(w394) -> ("RTG Ref"=w395:refnum<class "NI-RTG Interface.lvclass">, "Index"=w391:i32)
        n130 = call-dynamic "Send Target Configuration.vi"("error in"=w397, "target config"="Target Configuration", "device index (0)"=w391, "rtg api interface"=w395) -> ("error out"=w396:errorcluster, "rtg api interface out"=w392:refnum<class "NI-RTG Interface.lvclass">)  [unwired: 5 in, 1 out]
        n131 = Bundle By Name(cluster=w394, "RTG Ref"=w392) -> (w393:T16)
      }
      frame "RTG_Send Files" {
        # "----------------------------------20----------------------------------"
        # "21"
        n132 = Unbundle By Name(w412) -> ("AutoSend"=w400:bool, "Prepend"=w399:bool, "RTG Ref"=w401:refnum<class "NI-RTG Interface.lvclass">, "Index"=w402:i32)
        n133 = case shown="True" w399 {
          tunnel: w401 -> [w421 w426]
          tunnel: w405 -> [w420 w423]
          tunnel: w402 -> [_ w425]
          tunnel: [w421 w424] -> w406
          tunnel: [w420 w422] -> w410
          frame False {
          }
          frame True {
            # "requires software trigger"
            n134 = call-dynamic "Send Target Configuration.vi"("error in"=w423, "target config"=T6 {"synchronization"={"synch mode"=enum."Software Trigger", "time offset (s)"=0.0}, "rtg targets"=[{"time offset (s)"=0.0, "attenuaton (dB)"=0.0, "doppler"=0.0, "target enable"=FALSE, "relative velocity enable"=FALSE}, {"time offset (s)"=0.0, "attenuaton (dB)"=0.0, "doppler"=0.0, "target enable"=FALSE, "relative velocity enable"=FALSE}, {"time offset (s)"=0.0, "attenuaton (dB)"=0.0, "doppler"=0.0, "target enable"=FALSE, "relative velocity enable"=FALSE}, {"time offset (s)"=0.0, "attenuaton (dB)"=0.0, "doppler"=0.0, "target enable"=FALSE, "relative velocity enable"=FALSE}]}, "device index (0)"=w425, "rtg api interface"=w426) -> ("error out"=w422:errorcluster, "rtg api interface out"=w424:refnum<class "NI-RTG Interface.lvclass">)  [unwired: 5 in, 1 out]
          }
        }
        n135 = call-dynamic "Send Target Configuration List - Files.vi"("error in"=w410, "target configuration file path"="Target Configuration Files", "device index (0)"=w402, "rtg api interface"=w406) -> ("error out"=w409:errorcluster, "rtg api interface out"=w408:refnum<class "NI-RTG Interface.lvclass">)  [unwired: 6 in]
        n136 = case shown="True" w400 {
          tunnel: w408 -> [w414 w419]
          tunnel: [w414 w418] -> w403
          tunnel: w409 -> [w413 w417]
          tunnel: [w413 w416] -> w404
          tunnel: w402 -> [_ w415]
          frame False {
          }
          frame True {
            n137 = call-dynamic "Send Software Trigger.vi"("error in"=w417, "device index (0)"=w415, "NI-RTG Interface in"=w419) -> ("error out"=w416:errorcluster, "NI-RTG Interface out"=w418:refnum<class "NI-RTG Interface.lvclass">)  [unwired: 7 in]
          }
        }
        n138 = Bundle By Name(cluster=w412, "RTG Ref"=w403) -> (w411:T16)
      }
      frame "RTG_Send Motion" {
        # "----------------------------22----------------------------"
        n139 = Unbundle By Name(w441) -> ("AutoSend"=w428:bool, "Prepend"=w429:bool, "RTG Ref"=w431:refnum<class "NI-RTG Interface.lvclass">, "Index"=w430:i32)
        n140 = case shown="True" w429 {
          tunnel: w431 -> [w450 w455]
          tunnel: w434 -> [w449 w452]
          tunnel: w430 -> [_ w454]
          tunnel: [w450 w453] -> w435
          tunnel: [w449 w451] -> w439
          frame False {
          }
          frame True {
            # "requires software trigger"
            n141 = call-dynamic "Send Target Configuration.vi"("error in"=w452, "target config"=T6 {"synchronization"={"synch mode"=enum."Software Trigger", "time offset (s)"=0.0}, "rtg targets"=[{"time offset (s)"=0.0, "attenuaton (dB)"=0.0, "doppler"=0.0, "target enable"=FALSE, "relative velocity enable"=FALSE}, {"time offset (s)"=0.0, "attenuaton (dB)"=0.0, "doppler"=0.0, "target enable"=FALSE, "relative velocity enable"=FALSE}, {"time offset (s)"=0.0, "attenuaton (dB)"=0.0, "doppler"=0.0, "target enable"=FALSE, "relative velocity enable"=FALSE}, {"time offset (s)"=0.0, "attenuaton (dB)"=0.0, "doppler"=0.0, "target enable"=FALSE, "relative velocity enable"=FALSE}]}, "device index (0)"=w454, "rtg api interface"=w455) -> ("error out"=w451:errorcluster, "rtg api interface out"=w453:refnum<class "NI-RTG Interface.lvclass">)  [unwired: 5 in, 1 out]
          }
        }
        n142 = call-dynamic "Send Target Configuration List - Target Motion.vi"("error in"=w439, "target motion parameters"="Target Motion Parameters", "device index (0)"=w430, "rtg api interface"=w435) -> ("error out"=w437:errorcluster, "rtg api interface out"=w436:refnum<class "NI-RTG Interface.lvclass">)  [unwired: 6 in]
        n143 = case shown="True" w428 {
          tunnel: w436 -> [w443 w448]
          tunnel: [w443 w447] -> w432
          tunnel: w437 -> [w442 w446]
          tunnel: [w442 w445] -> w433
          tunnel: w430 -> [_ w444]
          frame False {
          }
          frame True {
            n144 = call-dynamic "Send Software Trigger.vi"("error in"=w446, "device index (0)"=w444, "NI-RTG Interface in"=w448) -> ("error out"=w445:errorcluster, "NI-RTG Interface out"=w447:refnum<class "NI-RTG Interface.lvclass">)  [unwired: 7 in]
          }
        }
        n145 = Bundle By Name(cluster=w441, "RTG Ref"=w432) -> (w440:T16)
      }
      frame "RTG_Send SW Trigg" {
        n146 = Unbundle By Name(w463) -> ("RTG Ref"=w458:refnum<class "NI-RTG Interface.lvclass">, "Index"=w459:i32)
        n147 = call-dynamic "Send Software Trigger.vi"("error in"=w461, "device index (0)"=w459, "NI-RTG Interface in"=w458) -> ("error out"=w460:errorcluster, "NI-RTG Interface out"=w457:refnum<class "NI-RTG Interface.lvclass">)  [unwired: 7 in]
        n148 = Bundle By Name(cluster=w463, "RTG Ref"=w457) -> (w462:T16)
      }
      frame "RTG_Chk" {
        n149 = Wait Until Next ms Multiple(millisecond multiple=u32 100) -> ()  [unwired: 1 out]
        n150 = Enqueue Element(queue=w472, element=cluster{"Enum":T3, "Var":variant} {"Enum"=enum."RTG_Chk", "Var"=variant}, error in (no error)=w473) -> (error out=w474:errorcluster)  [unwired: 1 in, 2 out]
        n151 = Unbundle By Name(w478) -> ("RTG Ref"=w475:refnum<class "NI-RTG Interface.lvclass">)
        n152 = call-dynamic "Get Coprocessor Link Status.vi"("error in"=w474, "rtg api interface"=w475) -> ("error out"=w468:errorcluster, "rtg link status"=→"rtg link status":T12[], "rtg api interface out"=w466:refnum<class "NI-RTG Interface.lvclass">)  [unwired: 7 in]
        n153 = call-dynamic "Get RTG Status.vi"("error in"=w468, "rtg api interface"=w466) -> ("error out"=w467:errorcluster, "rtg status"=→"RTG Status":string, "state"=w464:T13, "rtg api interface out"=w465:refnum<class "NI-RTG Interface.lvclass">)  [unwired: 6 in]
        "RTG State" <- w464
        n154 = Bundle By Name(cluster=w478, "RTG Ref"=w465, "state"=w464) -> (w477:T16)
      }
      frame "RTG_Exit" {
        # "RTG Exit is called from Coprocesor Exit\nto prevent a race condition"
        n155 = Unbundle By Name(w480) -> ("RTG Ref"=w481:refnum<class "NI-RTG Interface.lvclass">)
        n156 = call-dynamic "Close.vi"("error in"=w483, "rtg api interface"=w481) -> ("error out"=w484:errorcluster, "rtg api interface out"=w485:refnum<class "NI-RTG Interface.lvclass">)  [unwired: 8 in]
        n157 = call-dynamic "Destroy.vi"("error in"=w484, "NI-RTG Interface in"=w485) -> ("error out"=w482:errorcluster)  [unwired: 9 in]
      }
    }
    n158 = call "Log_Errors_20190313.vi"("LoopName"="RTG", "error in"=w148) -> ("error out"=w147:errorcluster)  [unwired: 9 in]
    "RTG" <- w144
  }
  n159 = while {
    tunnel: w20 -> [w488]
    tunnel: w1 -> [w486]
    stop <- w487 stop-if-true
    # "Event Loop"
    n160 = event shown="[2] \"Commit HW\": Value Change" {
      selector: _ -> [_ _ _ _ _ _ _ _ _ _]
      dyn-events: _ -> [_ _ _ _ _ _ _ _ _ _]
      timeout: 200 -> [_ _ _ _ _ _ _ _ _ _]
      tunnel: w488 -> [_ _ w495 _ _ _ _ _ _ w524]
      tunnel: [_ _ _ _ _ _ _ _ _ TRUE] -> w487
      tunnel: w486 -> [_ w492 _ w500 w504 w508 w512 w516 w520 _]
      event Timeout {
        n161 = event-data() -> ()  [unwired: 1 in, 3 out]
        n162 = Get Date/Time String() -> (time string=→"System Time":string)  [unwired: 3 in, 1 out]
      }
      event "Start RTG": Value Change {
        n163 = event-data() -> ()  [unwired: 1 in, 6 out]
        n164 = Enqueue Element(queue=w492, element=cluster{"Enum":T3, "Var":variant} {"Enum"=enum."RTG_Start", "Var"=variant}) -> (error out=w493:errorcluster)  [unwired: 2 in, 2 out]
        n165 = call "Log_Errors_20190313.vi"("LoopName"="EventStart", "error in"=w493) -> ()  [unwired: 9 in, 1 out]
      }
      event "Commit HW": Value Change {
        n166 = event-data() -> ()  [unwired: 1 in, 6 out]
        n167 = Enqueue Element(queue=w495, element=cluster{"Enum":T1, "Var":variant} {"Enum"=enum."Spvsr_InitRTG", "Var"=variant}) -> (error out=w497:errorcluster)  [unwired: 2 in, 2 out]
        n168 = call "Log_Errors_20190313.vi"("LoopName"="EventStart", "error in"=w497) -> ()  [unwired: 9 in, 1 out]
      }
      event "Send SW Trigg": Value Change {
        n169 = event-data() -> ()  [unwired: 1 in, 6 out]
        n170 = Enqueue Element(queue=w500, element=cluster{"Enum":T3, "Var":variant} {"Enum"=enum."RTG_Send SW Trigg", "Var"=variant}) -> (error out=w501:errorcluster)  [unwired: 2 in, 2 out]
        n171 = call "Log_Errors_20190313.vi"("LoopName"="SW_Trigg", "error in"=w501) -> ()  [unwired: 9 in, 1 out]
      }
      event "Stop RTG": Value Change {
        n172 = event-data() -> ()  [unwired: 1 in, 6 out]
        n173 = Enqueue Element(queue=w504, element=cluster{"Enum":T3, "Var":variant} {"Enum"=enum."RTG_Stop", "Var"=variant}) -> (error out=w505:errorcluster)  [unwired: 2 in, 2 out]
        n174 = call "Log_Errors_20190313.vi"("LoopName"="EventStop", "error in"=w505) -> ()  [unwired: 9 in, 1 out]
      }
      event "Device Index", "Prepend Software Trigger", "Auto Send Software Trigger": Value Change {
        n175 = event-data() -> ()  [unwired: 1 in, 6 out]
        n176 = Enqueue Element(queue=w508, element=cluster{"Enum":T3, "Var":variant} {"Enum"=enum."RTG_TargetSetup", "Var"=variant}) -> (error out=w509:errorcluster)  [unwired: 2 in, 2 out]
        n177 = call "Log_Errors_20190313.vi"("LoopName"="DevIndex", "error in"=w509) -> ()  [unwired: 9 in, 1 out]
      }
      event "Send TrgtCfg": Value Change {
        n178 = event-data() -> ()  [unwired: 1 in, 6 out]
        n179 = Enqueue Element(queue=w512, element=cluster{"Enum":T3, "Var":variant} {"Enum"=enum."RTG_Send Target Cfg", "Var"=variant}) -> (error out=w513:errorcluster)  [unwired: 2 in, 2 out]
        n180 = call "Log_Errors_20190313.vi"("LoopName"="SendTargetCfg", "error in"=w513) -> ()  [unwired: 9 in, 1 out]
      }
      event "Send Motion": Value Change {
        n181 = event-data() -> ()  [unwired: 1 in, 6 out]
        n182 = Enqueue Element(queue=w516, element=cluster{"Enum":T3, "Var":variant} {"Enum"=enum."RTG_Send Motion", "Var"=variant}) -> (error out=w517:errorcluster)  [unwired: 2 in, 2 out]
        n183 = call "Log_Errors_20190313.vi"("LoopName"="SendMotion", "error in"=w517) -> ()  [unwired: 9 in, 1 out]
      }
      event "Send Files": Value Change {
        n184 = event-data() -> ()  [unwired: 1 in, 6 out]
        n185 = Enqueue Element(queue=w520, element=cluster{"Enum":T3, "Var":variant} {"Enum"=enum."RTG_Send Files", "Var"=variant}) -> (error out=w521:errorcluster)  [unwired: 2 in, 2 out]
        n186 = call "Log_Errors_20190313.vi"("LoopName"="SendFiles", "error in"=w521) -> ()  [unwired: 9 in, 1 out]
      }
      event "Exit": Value Change {
        n187 = event-data() -> ()  [unwired: 1 in, 6 out]
        n188 = To Variant(anything=Program_Status_Enum."Closing" ("Status")) -> (Variant=w525:variant)
        n189 = Bundle By Name(cluster=cluster{"Enum":T1, "Var":variant} {"Enum"=enum."Spvsr_UpdtFP", "Var"=variant}, "Var"=w525) -> (w527:cluster{"Enum":T1, "Var":variant})
        n190 = Enqueue Element(queue=w524, element=w527) -> (queue out=w523:refnum<queue>)  [unwired: 2 in, 2 out]
        n191 = Enqueue Element(queue=w523, element=cluster{"Enum":T1, "Var":variant} {"Enum"=enum."Spvsr_Exit", "Var"=variant}) -> (error out=w530:errorcluster)  [unwired: 2 in, 2 out]
        n192 = call "Log_Errors_20190313.vi"("LoopName"="EventExit", "error in"=w530) -> ()  [unwired: 9 in, 1 out]
      }
    }
  }
  n193 = while {
    tunnel: w12 -> [w545]
    tunnel: [w547] -> w4
    tunnel: w2 -> [w544]
    tunnel: w1 -> [w541]
    tunnel: w20 -> [w534]
    shift-right: [w540] -> _
    shift-left: T15 {"CoPr Refs"=[]} -> [w539]
    i -> [w533]
    stop <- w535 stop-if-true
    # "CoProcessor Loop"
    n194 = Dequeue Element(queue=w544, error in (no error)=w545) -> (queue out=w536:refnum<queue>, element=w546:cluster{"Enum":T2, "Data":variant}, error out=w538:errorcluster)  [unwired: 1 in, 1 out]
    n195 = Unbundle(w546) -> ("Enum"=w543:T2, "Data"=w542:variant)
    "CoPr" <- w543
    n196 = case shown="\"CoPr_Chk\"" w543 {
      tunnel: w542 -> [w562 _ _]
      tunnel: w541 -> [w557 _ w619]
      tunnel: [w566 w582 w622] -> w540
      tunnel: w539 -> [w565 w582 w622]
      tunnel: w538 -> [w563 w591 w617]
      tunnel: [w558 w580 w624] -> w537
      tunnel: w536 -> [_ w590 _]
      tunnel: [_ _ TRUE] -> w535
      tunnel: w534 -> [_ w579 _]
      frame "CoPr_Init" {
        # "3. Create and Intialize Coprocessor Object if valid Coprocessor Hardware"
        # "3"
        n197 = Variant To Data(error in=w563, type="" ("option string"), Variant=w562) -> (data=w560:string, error out=w564:errorcluster)
        n198 = call <vilib>:"Create Coprocessor.vi"("error in"=w564, "option string"=w560, "coprocessor resources"="Coprocessor Names") -> ("error out"=w559:errorcluster, "rtg coprocessor links"=w554:refnum<class "RTG Coprocessor Link Interface.lvclass">[])  [unwired: 7 in]
        n199 = Bundle By Name(cluster=w565, "CoPr Refs"=w554) -> (w566:T15)
        n200 = To Variant(anything=w554) -> (Variant=w553:variant)
        n201 = Bundle By Name(cluster=cluster{"Enum":T3, "Var":variant} {"Enum"=enum."RTG_RefLvl", "Var"=variant}, "Var"=w553) -> (w555:cluster{"Enum":T3, "Var":variant})
        n202 = Build Array(w555, cluster{"Enum":T3, "Var":variant} {"Enum"=enum."RTG_mmWav", "Var"=variant}, cluster{"Enum":T3, "Var":variant} {"Enum"=enum."RTG_Cal", "Var"=variant}, cluster{"Enum":T3, "Var":variant} {"Enum"=enum."RTG_CalDone?", "Var"=variant}) -> (w552:cluster{"Enum":T3, "Var":variant}[])
        n203 = for {
          tunnel: w557 -> [w569]
          tunnel: w552 -> [w568] mode=indexing
          shift-right: [w570] -> w558
          shift-left: w559 -> [w571]
          n204 = Enqueue Element(queue=w569, element=w568, error in (no error)=w571) -> (error out=w570:errorcluster)  [unwired: 1 in, 2 out]
        }
      }
      frame "CoPr_Chk" {
        # "Send count\nwhen it \nchanges"
        n205 = Unbundle By Name(w582) -> ("CoPr Refs"=w583:refnum<class "RTG Coprocessor Link Interface.lvclass">[])
        n206 = Wait Until Next ms Multiple(millisecond multiple=u32 100) -> ()  [unwired: 1 out]
        n207 = Enqueue Element(queue=w590, element=cluster{"Enum":T2, "Data":variant} {"Enum"=enum."CoPr_Chk", "Data"=variant}, error in (no error)=w591) -> (error out=w584:errorcluster)  [unwired: 1 in, 2 out]
        n208 = for {
          tunnel: w583 -> [w604] mode=indexing
          tunnel: [w608] -> w585 mode=indexing
          shift-right: [w601] -> w581
          shift-left: w584 -> [w609]
          tunnel: [w603] -> w587 mode=indexing
          tunnel: [w597] -> w586 mode=indexing
          n209 = call-dynamic "Get Coprocessor Refnum.vi"("rtg coprocessor link interface"=w604) -> ("error out"=w607:errorcluster, "coprocessor refnum"=w605:refnum<k20>)  [unwired: 8 in, 1 out]
          n210 = call-dynamic "Coprocessor Link Status.vi"("error in"=w609, "rtg coprocessor link interface"=w604) -> ("error out"=w599:errorcluster, "coprocessor status out"=w608:T14, "rtg coprocessor link interface out"=w600:refnum<class "RTG Coprocessor Link Interface.lvclass">)  [unwired: 7 in]
          n211 = Not A Number/Path/Refnum?(number/path/refnum=w605) -> (NaN/Path/Refnum?=w606:bool)
          n212 = case shown="False" w606 {
            tunnel: w605 -> [w613 _]
            tunnel: w607 -> [w612 w616]
            tunnel: [w611 w616] -> w602
            tunnel: [w610 _] -> w603
            frame False {
              # "Read RTG coprocessor \nrecieved trigger count"
              n213 = Dynamic FPGA Interface Cast(Session In=refnum<k20> refnum ("Type"), Type=w613) -> (Session Out=w615:refnum<k20>)
              n214 = xnode "Read/Write Control"("FPGA VI Reference In"=w615, "error in"=w612) -> ("error out"=w611:errorcluster, "read trigger rising edge count"=w610:u16)  [unwired: 1 out]
            }
            frame True {
            }
          }
          n215 = call-dynamic "Get Device Index.vi"("error in"=w599, "rtg coprocessor link interface"=w600) -> ("error out"=w598:errorcluster, "device index"=w597:i32)  [unwired: 7 in, 1 out]
          n216 = Merge Errors(w598, w602) -> (w601:errorcluster)
        }
        "coproc link" <- w585
        n217 = Build Array(w586, w587) -> (w573:i32[][])
        n218 = feedback-in #1(w573) -> ()
        n219 = feedback #1(i32[][] []) -> (w574:i32[][])
        n220 = To Variant(anything=w573) -> (Variant=w576:variant)
        n221 = Not Equal?(x=w573, y=w574) -> (x != y?=w572:bool)
        n222 = Bundle By Name(cluster=cluster{"Enum":T1, "Var":variant} {"Enum"=enum."Spvsr_StateCount", "Var"=variant}, "Var"=w576) -> (w577:cluster{"Enum":T1, "Var":variant})
        n223 = case shown="True" w572 {
          tunnel: w581 -> [w592 w596]
          tunnel: [w592 w595] -> w580
          tunnel: w579 -> [_ w594]
          tunnel: w577 -> [_ w593]
          frame False {
          }
          frame True {
            n224 = Enqueue Element(queue=w594, element=w593, error in (no error)=w596) -> (error out=w595:errorcluster)  [unwired: 1 in, 2 out]
          }
        }
      }
      frame "CoPr_Exit" {
        n225 = Enqueue Element(queue=w619, element=cluster{"Enum":T3, "Var":variant} {"Enum"=enum."RTG_Exit", "Var"=variant}, error in (no error)=w617) -> (error out=w618:errorcluster)  [unwired: 1 in, 2 out]
        n226 = Unbundle By Name(w622) -> ("CoPr Refs"=w623:refnum<class "RTG Coprocessor Link Interface.lvclass">[])
        n227 = for {
          tunnel: w623 -> [w627] mode=indexing
          shift-right: [w625] -> w624
          shift-left: w618 -> [w626]
          # "29"
          n228 = call-dynamic "Close.vi"("error in"=w626, "rtg coprocessor link interface"=w627) -> ("error out"=w625:errorcluster)  [unwired: 9 in]
        }
      }
    }
    n229 = call "Log_Errors_20190313.vi"("LoopName"="CoPr", "error in"=w537) -> ("error out"=w547:errorcluster)  [unwired: 9 in]
    "CoPr" <- w533
  }
  n230 = flat-sequence {
    tunnel: w20 -> [w639]
    tunnel: w6 -> [w638]
    tunnel: w5 -> [w637]
    tunnel: w4 -> [w636]
    tunnel: w2 -> [w634]
    tunnel: w1 -> [w633]
    frame #0 {
      w632 = FALSE ("Stop RTG")
      n231 = Release Queue(queue=w639) -> (error out=w629:errorcluster)  [unwired: 2 in, 2 out]
      n232 = Release Queue(queue=w633) -> (error out=w630:errorcluster)  [unwired: 2 in, 2 out]
      n233 = Release Queue(queue=w634) -> (error out=w631:errorcluster)  [unwired: 2 in, 2 out]
      n234 = Merge Errors(w629, w630, w631, w638, w637, w636) -> (w635:errorcluster)
      n235 = local write "error out"(w635) -> ()
      n236 = local write "App Status"(Program_Status_Enum."Closed" ("App Status")) -> ()
      n237 = local write "Stop RTG"(w632) -> ()
      n238 = local write "Exit"(w632) -> ()
    }
  }
